vi "SetLengthTwenty.vi"(11 "Array_in(<20?)":i32[](array[numeric])) -> (3 "Array_out(n=20)":i32[](array[numeric]))   [LabVIEW 2014]
uses:
  <vilib>/Analysis/1siggen.llb/Riffle Array (I32).vi
  <vilib>/Analysis/NI_AALBase.lvlib
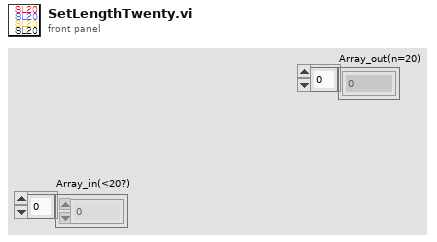
[diagram p1: front panel]
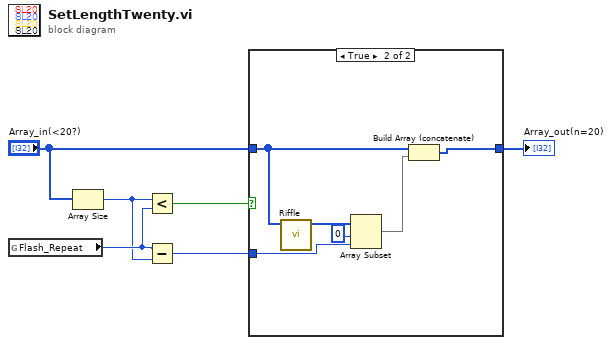
[diagram p0: block diagram]
diagram:
  n1 = global read "Control_Panel_정리.vi" "Flash_Repeat"() -> (w4:i32)
  n2 = Array Size(array="Array_in(<20?)") -> (size(s)=w3:i32)
  n3 = Less?(x=w3, y=w4) -> (x < y?=w6:bool)
  n4 = Subtract(x=w4, y=w3) -> (x-y=w2:i32)
  n5 = case shown="True" w6 {
    tunnel: "Array_in(<20?)" -> [w7 w10]
    tunnel: [w7 w8] -> w1
    tunnel: w2 -> [_ w12]
    frame False {
    }
    frame True {
      n6 = call-poly <vilib>:"Riffle.vi"("X"=w10) -> ("Riffled {X}"=w13:i32[])  [unwired: 8 in, 2 out]
      n7 = Array Subset(array=w13, index=0, length=w12) -> (w9:i32[])
      n8 = Build Array (concatenate)(w10, w9) -> (w8:i32[])
    }
  }
  "Array_out(n=20)" <- w1
